vi "exnSpectralBlock spectral measurements peak WFM (CDB).vi"(0 "Signals":waveform(cdb), 5 "Restart Averaging":bool, 7 "View":T2, 9 "Spectrum Window":u16, 11 "error in (no error)":errorcluster, 12 "Spectrum Averaging Parameters":T1={"averaging mode"=0, "weighting mode"=1, "number of averages"=10} {"averaging mode" items=["No averaging", "Vector averaging", "RMS averaging", "Peak hold"]; "weighting mode" items=["Linear", "Exponential"]}, 14 "All Spectra":bool) -> (4 "Measurement Output":cluster{"f0":dbl, "df":dbl, "magnitude":dbl[]}(graph), 6 "averaging done":bool, 10 "Phase":cluster{"f0":dbl, "df":dbl, "phase":dbl[]}(graph), 15 "error out":errorcluster)   [LabVIEW 2017]
uses:
  <vilib>/measure/NI_MAPro.lvlib
panel:
  in  "measurement":string="FFT - (Peak)"
  in  "string":string=" Phase"
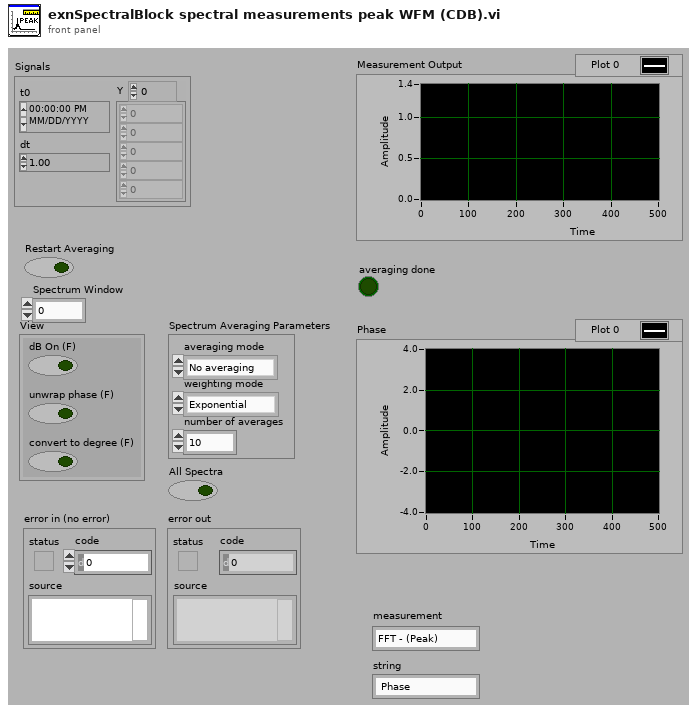
[diagram p1: front panel]
types:
  T1 = cluster{"averaging mode":u16, "weighting mode":u16, "number of averages":u32}
  T2 = cluster{"dB On (F)":bool, "unwrap phase (F)":bool, "convert to degree (F)":bool}
  T3 = enum16{"None ", "Hanning", "Hamming", "Blackman-Harris", "Exact Blackman", "Blackman", "Flat Top", "4 Term B-Harris ", "7 Term B-Harris", "Low Sidelobe"}
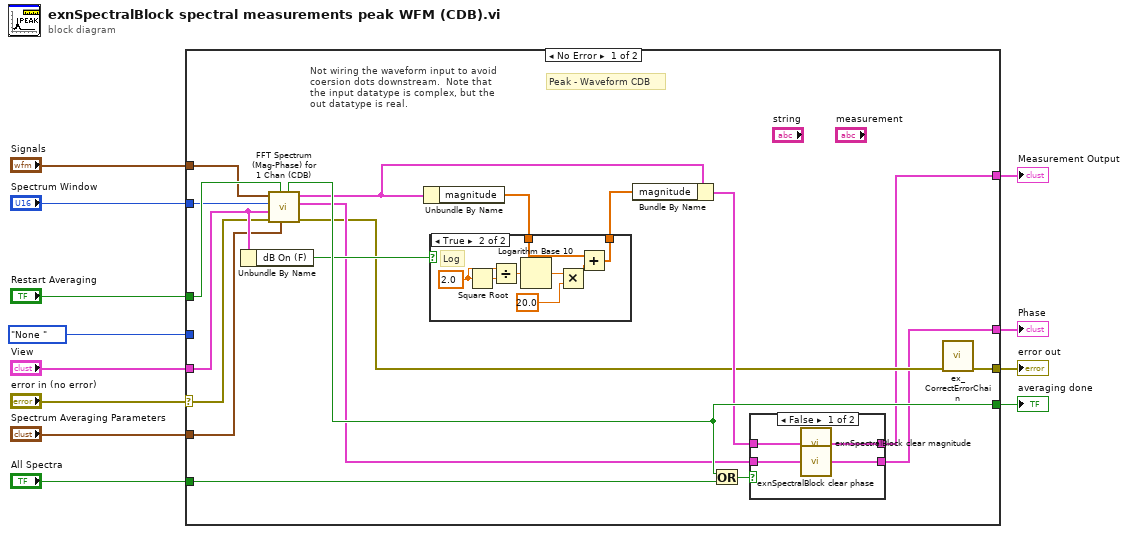
[diagram p0: block diagram]
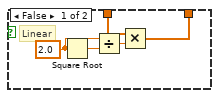
[diagram p2: hidden frame]
diagram:
  n1 = case shown="No Error" "error in (no error)" {
    selector: "error in (no error)" -> [w24 w51]
    tunnel: [w14 _] -> w12
    tunnel: [w13 _] -> w11
    tunnel: [w31 _] -> w10
    tunnel: "All Spectra" -> [w30 _]
    tunnel: "Spectrum Averaging Parameters" -> [w22 _]
    tunnel: "Restart Averaging" -> [w29 _]
    tunnel: T3."None " ("window") -> [_ _]
    tunnel: "Spectrum Window" -> [w25 _]
    tunnel: "View" -> [w28 _]
    tunnel: "Signals" -> [w20 _]
    tunnel: [w27 w51] -> w4
    frame No Error {
      # "Not wiring the waveform input to avoid coersion dots downstream.  Note that the input datatype is complex, but the out datatype is real."
      # "Peak - Waveform CDB"
      n2 = Unbundle By Name(w28) -> ("dB On (F)"=w23:bool)
      n3 = call <vilib>:"FFT Spectrum (Mag-Phase) for 1 Chan (CDB).vi"("averaging parameters"=w22, "restart averaging (F)"=w29, "error in (no error)"=w24, "view"=w28, "window"=w25, "time signal"=w20) -> ("error out"=w15:errorcluster, "phase"=w19:cluster{"f0":dbl, "df":dbl, "phase":dbl[]}, "magnitude"=w18:cluster{"f0":dbl, "df":dbl, "magnitude":dbl[]}, "averaging done"=w31:bool)  [unwired: 1 in, 1 out]
      n4 = Unbundle By Name(w18) -> ("magnitude"=w21:dbl[])
      n5 = case shown="True" w23 {
        tunnel: w21 -> [w35 w44]
        tunnel: [w34 w43] -> w17
        frame False {
          w33 = 2.0 ("y")
          # "Linear"
          n6 = Square Root(x=w33) -> (sqrt(x)=w36:dbl)
          n7 = Divide(x=w33, y=w36) -> (x/y=w32:dbl)
          n8 = Multiply(x=w35, y=w32) -> (x*y=w34:dbl[])
        }
        frame True {
          w41 = 2.0 ("y")
          # "Log"
          n9 = Square Root(x=w41) -> (sqrt(x)=w42:dbl)
          n10 = Divide(x=w41, y=w42) -> (x/y=w39:dbl)
          n11 = Logarithm Base 10(1:w39) -> (0:w37:dbl)
          n12 = Multiply(x=w37, y=20.0) -> (x*y=w38:dbl)
          n13 = Add(x=w44, y=w38) -> (x+y=w43:dbl[])
        }
      }
      n14 = Bundle By Name(cluster=w18, "magnitude"=w17) -> (w16:cluster{"f0":dbl, "df":dbl, "magnitude":dbl[]})
      n15 = Or(x=w31, y=w30) -> (x .or. y?=w26:bool)
      n16 = case shown="False" w26 {
        tunnel: w19 -> [w48 w49]
        tunnel: w16 -> [w46 w50]
        tunnel: [w45 w50] -> w14
        tunnel: [w47 w49] -> w13
        frame False {
          n17 = call <vilib>:"exnSpectralBlock clear magnitude.vi"("magnitude in"=w46) -> ("magnitude out"=w45:cluster{"f0":dbl, "df":dbl, "magnitude":dbl[]})
          n18 = call <vilib>:"exnSpectralBlock clear phase.vi"("phase in"=w48) -> ("phase out"=w47:cluster{"f0":dbl, "df":dbl, "phase":dbl[]})
        }
        frame True {
        }
      }
      n19 = call <vilib>:"ex_CorrectErrorChain.vi"("error in (no error)"=w15) -> ("error out"=w27:errorcluster)  [unwired: 10 in]
    }
    frame Error {
    }
  }
  "Phase" <- w11
  "Measurement Output" <- w12
  "averaging done" <- w10
  "error out" <- w4
